vi "Get Active Project.vi"(8 "error in (no error)":errorcluster) -> (0 "error out":errorcluster, 1 "No Active Project?":bool, 2 "Name":string, 3 "active project ref out":refnum<vi>)   [LabVIEW 2019, in "Configuration Tool.lvlib"]
uses:
  Configuration Tool.lvlib
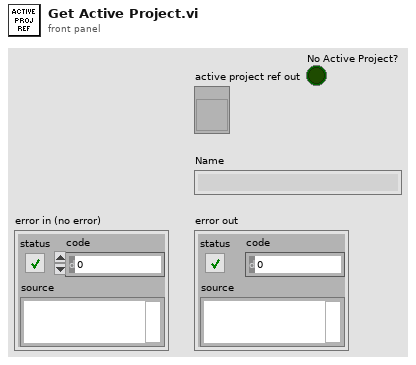
[diagram p1: front panel]
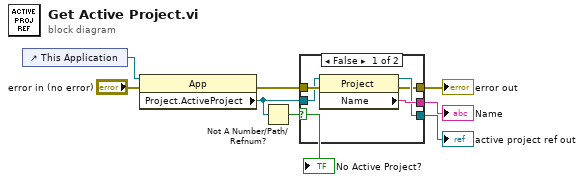
[diagram p0: block diagram]
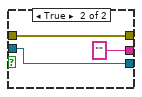
[diagram p2: hidden frame]
diagram:
  n1 = control-ref of="This Application"() -> (w8:refnum<vi>)
  n2 = property class="App"(reference=w8, error in="error in (no error)") -> (error out=w4:errorcluster, "Project.ActiveProject"=w2:refnum<vi>)  [unwired: 1 out]
  n3 = Not A Number/Path/Refnum?(number/path/refnum=w2) -> (NaN/Path/Refnum?=w1:bool)
  "No Active Project?" <- w1
  n4 = case shown="False" w1 {
    tunnel: [w13 "" ("Name")] -> w7
    tunnel: [w12 w16] -> w6
    tunnel: w4 -> [w11 w15]
    tunnel: [w10 w15] -> w3
    tunnel: w2 -> [w9 w16]
    frame False {
      n5 = property class="Project"(reference=w9, error in=w11) -> (reference out=w12:refnum<vi>, error out=w10:errorcluster, "Name"=w13:string)
    }
    frame True {
    }
  }
  "Name" <- w7
  "active project ref out" <- w6
  "error out" <- w3
